vi "Flatten Value.vi"(8 "Error In":errorcluster, 11 "Float In":refnum<class "Flt.lvclass">) -> (0 "Error Out":errorcluster, 1 "Value":string, 3 "Float Out":refnum<class "Flt.lvclass">)   [LabVIEW 2017, in "Tree API.lvlib" / "Flt.lvclass"]
uses:
  Flt.lvclass
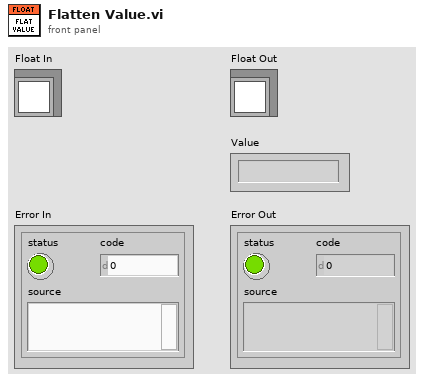
[diagram p1: front panel]
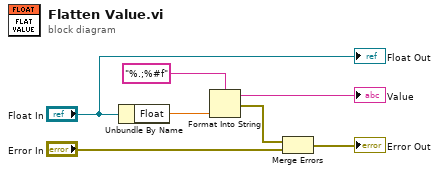
[diagram p0: block diagram]
diagram:
  n1 = Unbundle By Name("Float In") -> ("Float"=w3:dbl)
  n2 = Format Into String(format string="%.;%#f" ("initial string"), w3) -> (resulting string=→"Value":string, error out=w6:errorcluster)  [unwired: 2 in]
  n3 = Merge Errors(w6, "Error In") -> (→"Error Out":errorcluster)
  "Float Out" <- "Float In"
